vi "ZeroMQ_TCS.vi"() -> ()   [LabVIEW 2018]
uses:
  <vilib>/addons/zeromq/socket_type.ctl
  <vilib>/addons/zeromq/socket_options.ctl
  <vilib>/addons/zeromq/zeromq.lvlib
  <vilib>/addons/zeromq/zmq_socket.lvclass
  <vilib>/addons/zeromq/zmq_context.lvclass
panel:
  in  "stop 3":bool
  out "command":string
  out "error out 3":errorcluster
  out "message":string
  out "error out 2":errorcluster
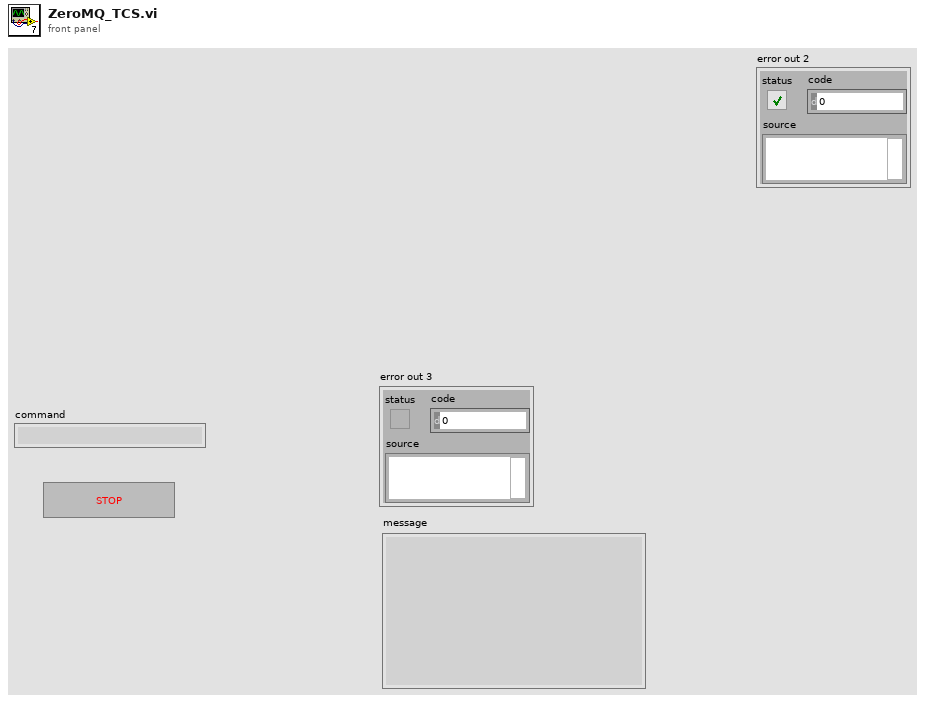
[diagram p1: front panel]
types:
  T1 = cluster{"ID":u32, "Address":string, "Service Name 1":string, "Service Name 2":string, "queue TX":refnum<queue>, "queue RX":refnum<queue>, "Port 1":u32, "Port 2":u32}
  T2 = typedef "zeromq.lvlib/socket_options.ctl" = enum8{"NONE", "ZMQ_HWM", "<2>", "ZMQ_SWAP", "ZMQ_AFFINITY", "ZMQ_ROUTING_ID", "ZMQ_SUBSCRIBE", "ZMQ_UNSUBSCRIBE", "ZMQ_RATE", "ZMQ_RECOVERY_IVL", "ZMQ_MCAST_LOOP", "ZMQ_SNDBUF", "ZMQ_RCVBUF", "ZMQ_RCVMORE", "ZMQ_FD", "ZMQ_EVENTS", "ZMQ_TYPE", "ZMQ_LINGER", "ZMQ_RECONNECT_IVL", "ZMQ_BACKLOG", "ZMQ_RECOVERY_IVL_MSEC", "ZMQ_RECONNECT_IVL_MAX", "ZMQ_MAXMSGSIZE", "ZMQ_SNDHWM", "ZMQ_RCVHWM", "ZMQ_MULTICAST_HOPS", "<26>", "ZMQ_RCVTIMEO", "ZMQ_SNDTIMEO", "<29>", "<30>", "ZMQ_IPV4ONLY", "ZMQ_LAST_ENDPOINT", "ZMQ_ROUTER_MANDATORY", "ZMQ_TCP_KEEPALIVE", "ZMQ_TCP_KEEPALIVE_CNT", "ZMQ_TCP_KEEPALIVE_IDLE", "ZMQ_TCP_KEEPALIVE_INTVL", "ZMQ_TCP_ACCEPT_FILTER", "ZMQ_IMMEDIATE", "ZMQ_XPUB_VERBOSE", "ZMQ_ROUTER_RAW", "ZMQ_IPV6", "ZMQ_MECHANISM", "ZMQ_PLAIN_SERVER", "ZMQ_PLAIN_USERNAME", "ZMQ_PLAIN_PASSWORD", "ZMQ_CURVE_SERVER", "ZMQ_CURVE_PUBLICKEY", "ZMQ_CURVE_SECRETKEY", "ZMQ_CURVE_SERVERKEY", "ZMQ_PROBE_ROUTER", "ZMQ_REQ_CORRELATE", "ZMQ_REQ_RELAXED", "ZMQ_CONFLATE", "ZMQ_ZAP_DOMAIN", "ZMQ_ROUTER_HANDOVER", "ZMQ_TOS", "ZMQ_IPC_FILTER_PID", "ZMQ_IPC_FILTER_UID", "ZMQ_IPC_FILTER_GID", "ZMQ_CONNECT_ROUTING_ID", "ZMQ_GSSAPI_SERVER", "ZMQ_GSSAPI_PRINCIPAL", "ZMQ_GSSAPI_SERVICE_PRINCIPAL", "ZMQ_GSSAPI_PLAINTEXT", "ZMQ_HANDSHAKE_IVL", "<67>", "ZMQ_SOCKS_PROXY", "ZMQ_XPUB_NODROP", "ZMQ_BLOCKY", "ZMQ_XPUB_MANUAL", "ZMQ_XPUB_WELCOME_MSG", "ZMQ_STREAM_NOTIFY", "ZMQ_INVERT_MATCHING", "ZMQ_HEARTBEAT_IVL", "ZMQ_HEARTBEAT_TTL", "ZMQ_HEARTBEAT_TIMEOUT", "ZMQ_XPUB_VERBOSER", "ZMQ_CONNECT_TIMEOUT", "ZMQ_TCP_MAXRT", "ZMQ_THREAD_SAFE", "<82>", "<83>", "ZMQ_MULTICAST_MAXTPDU", "ZMQ_VMCI_BUFFER_SIZE", "ZMQ_VMCI_BUFFER_MIN_SIZE", "ZMQ_VMCI_BUFFER_MAX_SIZE", "ZMQ_VMCI_CONNECT_TIMEOUT", "ZMQ_USE_FD", "ZMQ_GSSAPI_PRINCIPAL_NAMETYPE", "ZMQ_GSSAPI_SERVICE_PRINCIPAL_NAMETYPE", "ZMQ_BINDTODEVICE", "ZMQ_ZAP_ENFORCE_DOMAIN", "ZMQ_LOOPBACK_FASTPATH", "ZMQ_METADATA", "ZMQ_MULTICAST_LOOP", "ZMQ_ROUTER_NOTIFY"}
  T3 = typedef "zeromq.lvlib/socket_type.ctl" = enum8{"ZMQ_PAIR", "ZMQ_PUB", "ZMQ_SUB", "ZMQ_REQ", "ZMQ_REP", "ZMQ_DEALER", "ZMQ_ROUTER", "ZMQ_PULL", "ZMQ_PUSH", "ZMQ_XPUB", "ZMQ_XSUB", "ZMQ_STREAM", "ZMQ_SERVER", "ZMQ_CLIENT", "ZMQ_RADIO", "ZMQ_DISH", "ZMQ_GATHER", "ZMQ_SCATTER", "ZMQ_DGRAM"}
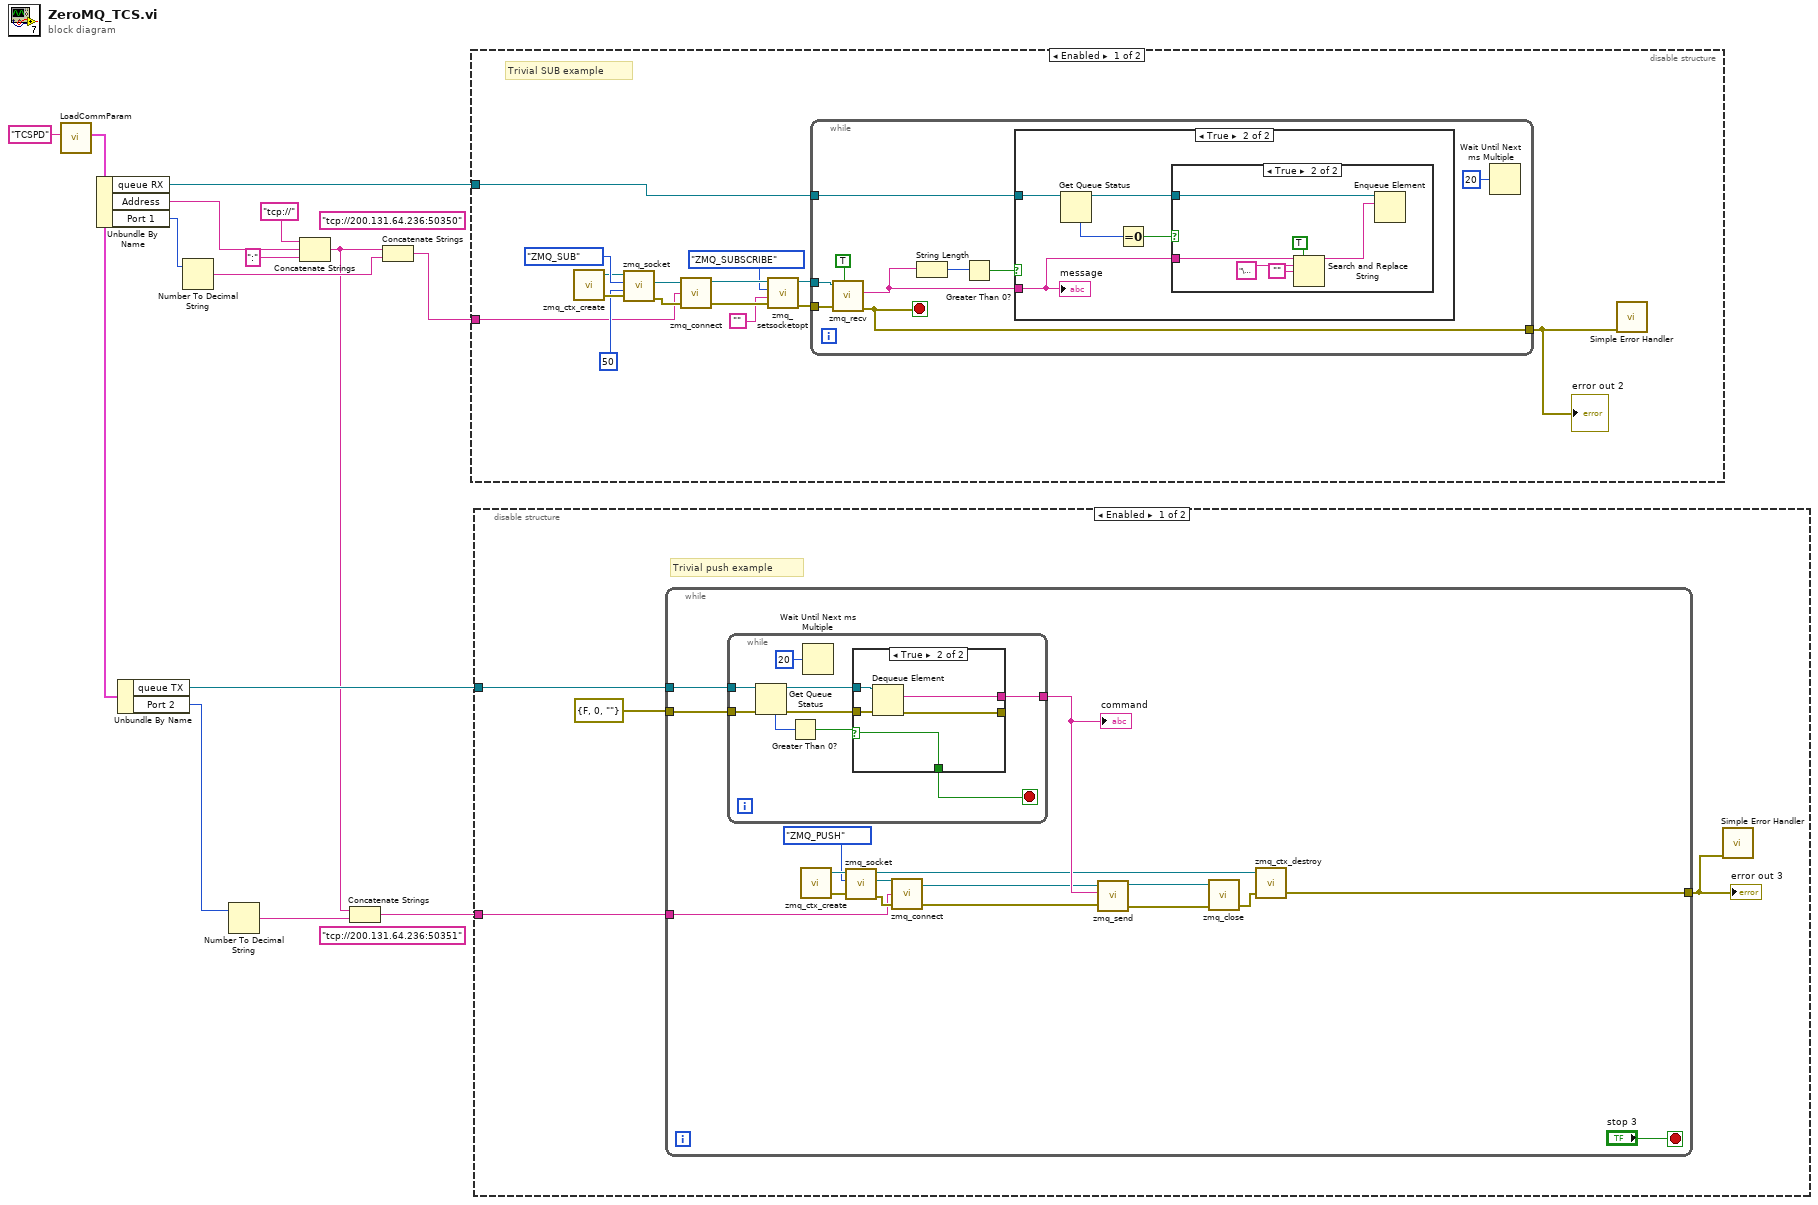
[diagram p0: block diagram]
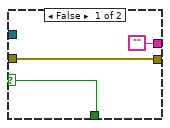
[diagram p2: hidden frame]
diagram:
  (unwired) "tcp://200.131.64.236:50351" ("endpoint")
  (unwired) "tcp://200.131.64.236:50350" ("endpoint")
  n1 = call "LoadCommParam.vi"("section name"="TCSPD") -> ("output cluster"=w7:T1)  [unwired: 10 in]
  n2 = Unbundle By Name(w7) -> ("queue RX"=w13:refnum<queue>, "Address"=w11:string, "Port 1"=w9:u32)
  n3 = Unbundle By Name(w7) -> ("queue TX"=w8:refnum<queue>, "Port 2"=w4:u32)
  n4 = Number To Decimal String(number=w9) -> (decimal integer string=w6:string)  [unwired: 1 in]
  n5 = Number To Decimal String(number=w4) -> (decimal integer string=w2:string)  [unwired: 1 in]
  n6 = Concatenate Strings("tcp://" ("string"), w11, ":" ("string")) -> (w3:string)
  n7 = Concatenate Strings(w3, w2) -> (w1:string)
  n8 = Concatenate Strings(w3, w6) -> (w5:string)
  n9 = disable-structure shown="Enabled" {
    disable-tunnel: w13 -> [w16 _]
    disable-tunnel: w5 -> [w15 _]
    frame Enabled {
      # "Trivial SUB example"
      n10 = call <vilib>:"zmq_ctx_create.vi"() -> ("error out"=w28:errorcluster, "context out"=w18:refnum<class "zmq_context.lvclass">)  [unwired: 4 in]
      n11 = call <vilib>:"zmq_socket.vi"("error in"=w28, "linger (ms)"=50, "socket type"=socket_type."ZMQ_SUB", "context in"=w18) -> ("error out"=w27:errorcluster, "socket out"=w19:refnum<class "zmq_socket.lvclass">)  [unwired: 1 in, 1 out]
      n12 = call <vilib>:"zmq_connect.vi"("error in"=w27, "endpoint"=w15, "socket in"=w19) -> ("error out"=w25:errorcluster, "socket out"=w26:refnum<class "zmq_socket.lvclass">)  [unwired: 1 in]
      n13 = call <vilib>:"zmq_setsocketopt.vi"("error in"=w25, "value"="", "option"=socket_options."ZMQ_SUBSCRIBE", "socket in"=w26) -> ("error out"=w24:errorcluster, "socket out"=w23:refnum<class "zmq_socket.lvclass">)  [unwired: 2 in]
      n14 = while {
        tunnel: w23 -> [w36]
        tunnel: w24 -> [w38]
        tunnel: [w37] -> w20
        tunnel: w16 -> [w33]
        stop <- w37 stop-if-true
        n15 = call <vilib>:"zmq_recv.vi"("no block? (F)"=TRUE, "error in"=w38, "socket in"=w36) -> ("error out"=w37:errorcluster, "data"=w32:string)  [unwired: 2 in, 3 out]
        n16 = String Length(string=w32) -> (length=w35:i32)
        n17 = Greater Than 0?(x=w35) -> (x > 0?=w34:bool)
        n18 = case shown="True" w34 {
          tunnel: w33 -> [_ w42]
          tunnel: w32 -> [_ w39]
          frame False {
          }
          frame True {
            n19 = Get Queue Status(queue=w42) -> (queue out=w40:refnum<queue>, # elements in queue=w43:i32)  [unwired: 2 in, 6 out]
            n20 = Equal To 0?(x=w43) -> (x = 0?=w41:bool)
            n21 = case shown="True" w41 {
              tunnel: w40 -> [_ w49]
              tunnel: w39 -> [_ w48]
              frame False {
              }
              frame True {
                n22 = Search and Replace String(replace all?=TRUE ("replace all? (F)"), input string=w48, search string="\u0000" ("substring (\"\")"), replace string="" ("replace string (\"\")")) -> (result string=w44:string)  [unwired: 4 in, 3 out]
                n23 = Enqueue Element(queue=w49, element=w44) -> ()  [unwired: 2 in, 3 out]
              }
            }
            "message" <- w39
          }
        }
        n24 = Wait Until Next ms Multiple(millisecond multiple=u32 20) -> ()  [unwired: 1 out]
      }
      "error out 2" <- w20
      n25 = call <vilib>:"Simple Error Handler.vi"("error in (no error)"=w20) -> ()  [unwired: 4 in, 5 out]
    }
    frame Disabled {
    }
  }
  n26 = disable-structure shown="Enabled" {
    disable-tunnel: w8 -> [w51 _]
    disable-tunnel: w1 -> [w50 _]
    frame Enabled {
      # "Trivial push example"
      n27 = while {
        tunnel: w51 -> [w70]
        tunnel: errorcluster {"status"=FALSE, "code"=0, "source"=""} ("error out") -> [w69]
        tunnel: [w58] -> w53
        tunnel: w50 -> [w54]
        stop <- "stop 3" stop-if-true
        n28 = while {
          tunnel: w70 -> [w78]
          tunnel: w69 -> [w77]
          tunnel: [w73] -> w68
          stop <- w72 stop-if-true
          n29 = Get Queue Status(queue=w78, error in (no error)=w77) -> (queue out=w74:refnum<queue>, error out=w75:errorcluster, # elements in queue=w79:i32)  [unwired: 1 in, 5 out]
          n30 = Greater Than 0?(x=w79) -> (x > 0?=w76:bool)
          n31 = Wait Until Next ms Multiple(millisecond multiple=u32 20) -> ()  [unwired: 1 out]
          n32 = case shown="True" w76 {
            selector: w76 -> [w80 w83]
            tunnel: w75 -> [w82 w87]
            tunnel: w74 -> [_ w86]
            tunnel: [w82 w85] -> _
            tunnel: ["" w84] -> w73
            tunnel: [w80 w83] -> w72
            frame False {
            }
            frame True {
              n33 = Dequeue Element(queue=w86, error in (no error)=w87) -> (element=w84:string, error out=w85:errorcluster)  [unwired: 1 in, 2 out]
            }
          }
        }
        "command" <- w68
        n34 = call <vilib>:"zmq_ctx_create.vi"() -> ("error out"=w63:errorcluster, "context out"=w66:refnum<class "zmq_context.lvclass">)  [unwired: 4 in]
        n35 = call <vilib>:"zmq_socket.vi"("error in"=w63, "socket type"=socket_type."ZMQ_PUSH", "context in"=w66) -> ("error out"=w65:errorcluster, "socket out"=w64:refnum<class "zmq_socket.lvclass">, "context out"=w57:refnum<class "zmq_context.lvclass">)  [unwired: 2 in]
        n36 = call <vilib>:"zmq_connect.vi"("error in"=w65, "endpoint"=w54, "socket in"=w64) -> ("error out"=w60:errorcluster, "socket out"=w61:refnum<class "zmq_socket.lvclass">)  [unwired: 1 in]
        n37 = call <vilib>:"zmq_send.vi"("error in"=w60, "data"=w68, "socket in"=w61) -> ("error out"=w55:errorcluster, "socket out"=w56:refnum<class "zmq_socket.lvclass">)  [unwired: 4 in]
        n38 = call <vilib>:"zmq_close.vi"("error in"=w55, "socket"=w56) -> ("error out"=w59:errorcluster)  [unwired: 3 in]
        n39 = call <vilib>:"zmq_ctx_destroy.vi"("error in"=w59, "context in"=w57) -> ("error out"=w58:errorcluster)  [unwired: 3 in]
      }
      "error out 3" <- w53
      n40 = call <vilib>:"Simple Error Handler.vi"("error in (no error)"=w53) -> ()  [unwired: 4 in, 5 out]
    }
    frame Disabled {
    }
  }
